vi "Nickname (Read).vi"(6 "ISOBUS address":T2=-1 caption="ISOBUS address (-1)", 8 "error in":errorcluster, 11 "Mercury Reference In":T3) -> (0 "error out":errorcluster, 2 "Nickname":string, 3 "Mercury Reference Out":T3, 4 "Valid?":T1)   [LabVIEW 2019, in "Mercury iXX.lvlib" / "Magnet.lvlib"]
doc: "Read the Nickname of the selected magnet PSU device."
uses:
  Magnet.lvlib
  Controls/Mercury Reference.ctl
  Controls/Comms Transport Layer.ctl
  Private/Controls/Query Dynamic Reference.ctl
  Controls/ISOBus Address.ctl
  Controls/Is Valid LED.ctl
  Private/Controls/Command Verbs.ctl
  Mercury iXX.lvlib
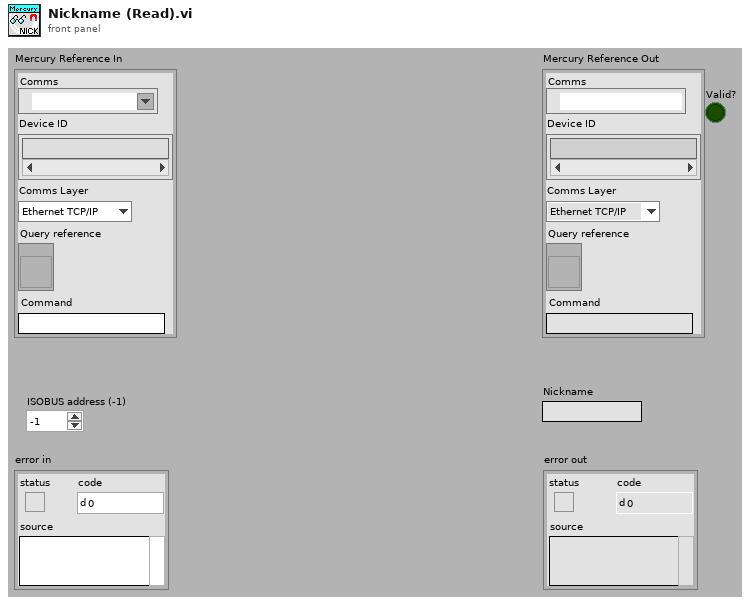
[diagram p1: front panel]
types:
  T1 = typedef "Mercury iXX.lvlib/Is Valid LED.ctl" = bool
  T2 = typedef "Mercury iXX.lvlib/ISOBus Address.ctl" = i32
  T3 = typedef "Mercury iXX.lvlib/Mercury Reference.ctl" = cluster{"Comms":refnum<visa-resource-name>, "Device ID":string[], "Comms Layer":T4, "Command":string, "Query reference":T5}
  T4 = typedef "Mercury iXX.lvlib/Comms Transport Layer.ctl" = enum16{"Ethernet TCP/IP", "USB", "ISOBus - RS-232", "GPIB"}
  T5 = typedef "Mercury iXX.lvlib/Query Dynamic Reference.ctl" = refnum<vi>
  T6 = typedef "Mercury iXX.lvlib/Command Verbs.ctl" = string
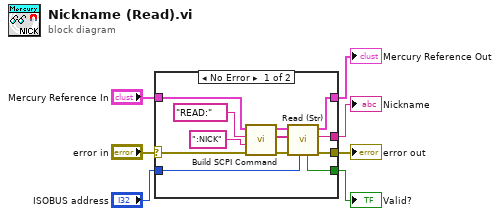
[diagram p0: block diagram]
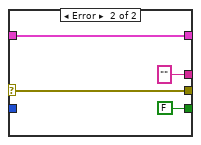
[diagram p2: hidden frame]
diagram:
  n1 = case shown="No Error" "error in" {
    selector: "error in" -> [w13 w22]
    tunnel: "Mercury Reference In" -> [w17 w23]
    tunnel: [w16 w23] -> w6
    tunnel: "ISOBUS address" -> [w10 _]
    tunnel: [w9 T1 FALSE ("Valid?")] -> w4
    tunnel: [w14 w22] -> w3
    tunnel: [w15 "" ("Response")] -> w2
    frame No Error {
      n2 = call "Build SCPI Command.vi"("error in"=w13, "Noun(s)"=":NICK" ("Command"), "Verb"=T6 "READ:", "Mercury Reference In"=w17) -> ("error out"=w11:errorcluster, "SCPI Message(s)"=w8:string[], "Mercury Reference Out"=w12:T3)  [unwired: 5 out]
      n3 = call "Read (Str).vi"("ISOBUS address"=w10, "error in"=w11, "SCPI Message(s)"=w8, "Mercury Reference In"=w12) -> ("error out"=w14:errorcluster, "Response"=w15:string, "Mercury Reference Out"=w16:T3, "Valid?"=w9:T1)  [unwired: 4 out]
    }
    frame Error {
    }
  }
  "Mercury Reference Out" <- w6
  "error out" <- w3
  "Valid?" <- w4
  "Nickname" <- w2
